vi "Make_Sequence.vi"() -> (3 "Sequence":T1)   [LabVIEW 2017]
doc: "SubVI que genera el nuevo elemento de la secuencia."
uses:
  Controls/Sequence.ctl
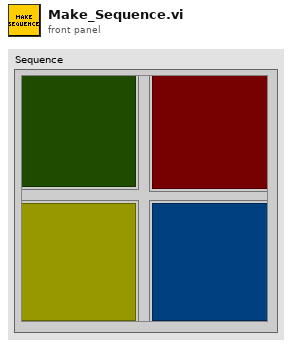
[diagram p1: front panel]
types:
  T1 = typedef "Sequence.ctl" = cluster{"S1":bool, "S2":bool, "S3":bool, "S4":bool}
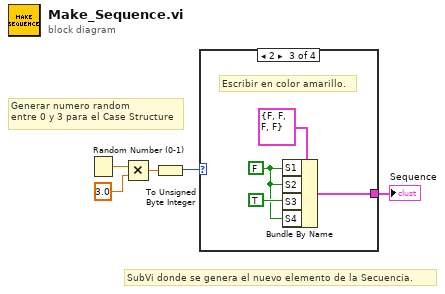
[diagram p0: block diagram]
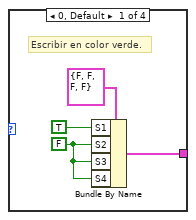
[diagram p2: hidden frame]
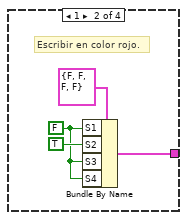
[diagram p3: hidden frame]
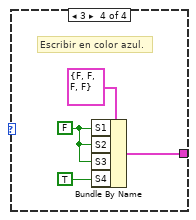
[diagram p4: hidden frame]
diagram:
  # "Generar numero random\nentre 0 y 3 para el Case Structure"
  # "SubVi donde se genera el nuevo elemento de la Secuencia."
  n1 = Random Number (0-1)() -> (number: 0 to 1=w5:dbl)
  n2 = Multiply(x=w5, y=3.0) -> (x*y=w3:dbl)
  n3 = To Unsigned Byte Integer(number=w3) -> (unsigned 8bit integer=w2:u8)
  n4 = case shown="2" w2 {
    tunnel: [w6 w10 w14 w18] -> w1
    frame 0, Default {
      w7 = FALSE ("S1")
      # "Escribir en color verde."
      n5 = Bundle By Name(cluster=T1 {"S1"=FALSE, "S2"=FALSE, "S3"=FALSE, "S4"=FALSE} ("Sequence"), "S1"=TRUE, "S2"=w7, "S3"=w7, "S4"=w7) -> (w6:T1)
    }
    frame 1 {
      w11 = FALSE ("S1")
      # "Escribir en color rojo."
      n6 = Bundle By Name(cluster=T1 {"S1"=FALSE, "S2"=FALSE, "S3"=FALSE, "S4"=FALSE} ("Sequence"), "S1"=w11, "S2"=TRUE ("S1"), "S3"=w11, "S4"=w11) -> (w10:T1)
    }
    frame 2 {
      w15 = FALSE ("S1")
      # "Escribir en color amarillo."
      n7 = Bundle By Name(cluster=T1 {"S1"=FALSE, "S2"=FALSE, "S3"=FALSE, "S4"=FALSE} ("Sequence"), "S1"=w15, "S2"=w15, "S3"=TRUE ("S1"), "S4"=w15) -> (w14:T1)
    }
    frame 3 {
      w19 = FALSE ("S1")
      # "Escribir en color azul."
      n8 = Bundle By Name(cluster=T1 {"S1"=FALSE, "S2"=FALSE, "S3"=FALSE, "S4"=FALSE} ("Sequence"), "S1"=w19, "S2"=w19, "S3"=w19, "S4"=TRUE ("S1")) -> (w18:T1)
    }
  }
  "Sequence" <- w1
